vi "DesiredRow2DesiredBundle.vi"(0 "DesiredStatRow":string[](array[string])) -> (4 "DesiredParameters":T1, 8 "Controller?":bool)   [LabVIEW 2013]
uses:
  TypeDef/Command Cluster.ctl
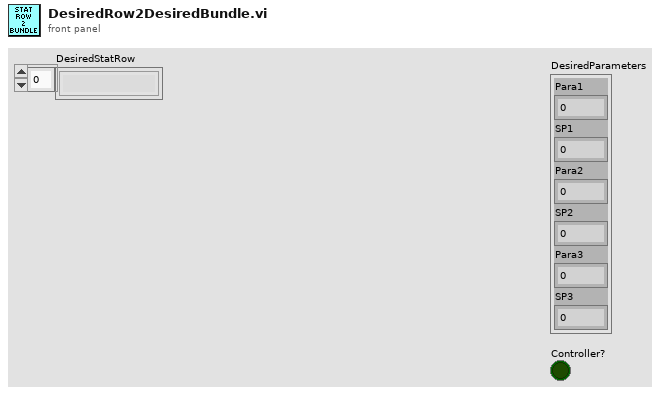
[diagram p1: front panel]
types:
  T1 = typedef "Command Cluster.ctl" = cluster{"Para1":i32, "SP1":dbl, "Para2":i32, "SP2":dbl, "Para3":i32, "SP3":dbl}
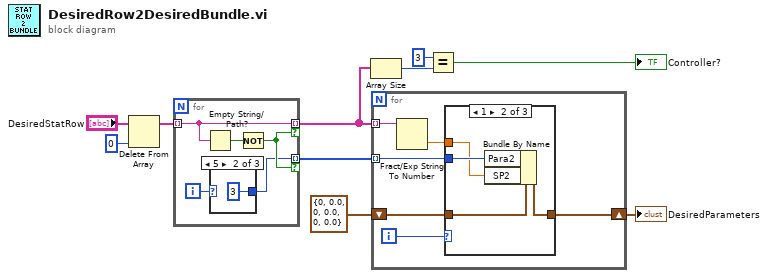
[diagram p0: block diagram]
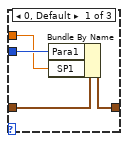
[diagram p2: hidden frame]
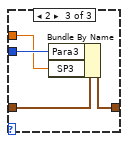
[diagram p3: hidden frame]
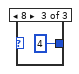
[diagram p5: hidden frame]
diagram:
  n1 = Delete From Array(array="DesiredStatRow", index=0) -> (array with subset deleted=w8:string[])  [unwired: 1 in, 1 out]
  n2 = for {
    tunnel: w8 -> [w15] mode=indexing
    tunnel: [w15] -> w7 mode=indexing if=w13
    tunnel: [w11] -> w6 mode=indexing if=w13
    i -> [w12]
    n3 = Empty String/Path?(string/path=w15) -> (empty?=w14:bool)
    n4 = case shown="5" w12 {
      selector: w12 -> [w16 _ _]
      tunnel: [w16 3 4] -> w11
      frame 0..2, Default {
      }
      frame 5 {
      }
      frame 8 {
      }
    }
    n5 = Not(x=w14) -> (.not. x?=w13:bool)
  }
  n6 = Array Size(array=w7) -> (size(s)=w5:i32)
  n7 = for {
    tunnel: w7 -> [w20] mode=indexing
    tunnel: w6 -> [w21] mode=indexing
    shift-right: [w22] -> w1
    shift-left: T1 {"Para1"=0, "SP1"=0.0, "Para2"=0, "SP2"=0.0, "Para3"=0, "SP3"=0.0} ("DesiredParameters") -> [w23]
    i -> [w24]
    n8 = Fract/Exp String To Number(string=w20) -> (number=w19:dbl)  [unwired: 3 in, 1 out]
    n9 = case shown="1" w24 {
      tunnel: w23 -> [w28 w32 w36]
      tunnel: [w27 w31 w35] -> w22
      tunnel: w21 -> [w26 w30 w34]
      tunnel: w19 -> [w25 w29 w33]
      frame 0, Default {
        n10 = Bundle By Name(cluster=w28, "Para1"=w26, "SP1"=w25) -> (w27:T1)
      }
      frame 1 {
        n11 = Bundle By Name(cluster=w32, "Para2"=w30, "SP2"=w29) -> (w31:T1)
      }
      frame 2 {
        n12 = Bundle By Name(cluster=w36, "Para3"=w34, "SP3"=w33) -> (w35:T1)
      }
    }
  }
  "DesiredParameters" <- w1
  n13 = Equal?(x=3, y=w5) -> (x = y?=→"Controller?":bool)
